vi "StatorResistanceEstimation.vi"(11 "nameplate information":T1) -> (3 "stator resisitance [ohms]":dbl)   [LabVIEW 2017, in "McsaAnalysisFunctions.lvlib"]
doc: "Estimates motor stator resistance based on nameplate information."
uses:
  <vilib>/addons/InsightCM/Utilities/Analysis/MCSA/McsaAnalysisFunctions.lvlib
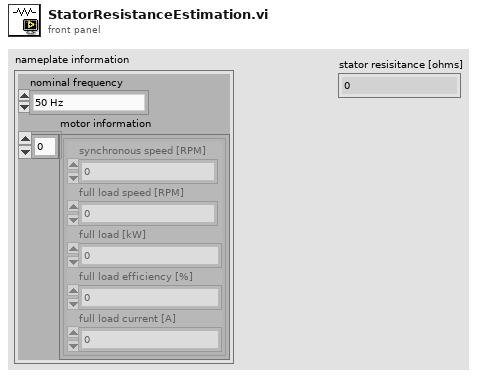
[diagram p1: front panel]
types:
  T1 = cluster{"nominal frequency":enum16{"50 Hz", "60 Hz"}, "motor information":cluster{"synchronous speed [RPM]":dbl, "full load speed [RPM]":dbl, "full load [kW]":dbl, "full load efficiency [%]":dbl, "full load current [A]":dbl}[]}
  T2 = cluster{"synchronous speed [RPM]":dbl, "full load speed [RPM]":dbl, "full load [kW]":dbl, "full load efficiency [%]":dbl, "full load current [A]":dbl}[]
  T3 = cluster{"synchronous speed [RPM]":dbl, "full load speed [RPM]":dbl, "full load [kW]":dbl, "full load efficiency [%]":dbl, "full load current [A]":dbl}
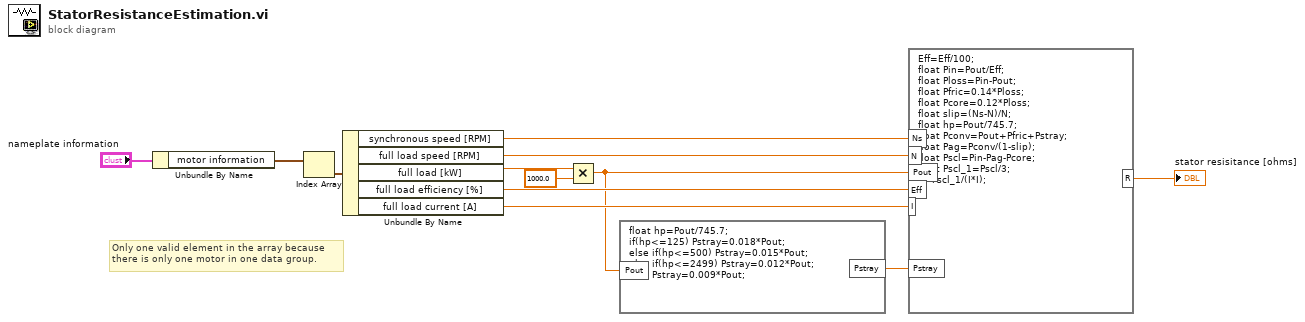
[diagram p0: block diagram]
diagram:
  # "Only one valid element in the array because\nthere is only one motor in one data group."
  n1 = Unbundle By Name("nameplate information") -> ("motor information"=w3:T2)
  n2 = Index Array(array=w3) -> (element=w2:T3)  [unwired: 1 in]
  n3 = Unbundle By Name(w2) -> ("synchronous speed [RPM]"=w10:dbl, "full load speed [RPM]"=w9:dbl, "full load [kW]"=w11:dbl, "full load efficiency [%]"=w6:dbl, "full load current [A]"=w8:dbl)
  n4 = Multiply(x=w11, y=1000.0) -> (x*y=w5:dbl)
  n5 = formula code="float hp=Pout/745.7;\nif(hp<=125) Pstray=0.018*Pout;\nelse if(hp<=500) Pstray=0.015*Pout;\nelse if(hp<=2499) Pstray=0.012*Pout;\nelse Pstray=0.009*Pout;"("Pout"=w5) -> ("Pstray"=w7:dbl)
  n6 = formula code="Eff=Eff/100;\nfloat Pin=Pout/Eff;\nfloat Ploss=Pin-Pout;\nfloat Pfric=0.14*Ploss;\nfloat Pcore=0.12*Ploss;\nfloat slip=(Ns-N)/N;\nfloat hp=Pout/745.7;\nfloat Pconv=Pout+Pfric+Pstray;\nfloat Pag=Pconv/(1-slip);\nfloat Pscl=Pin-Pag-Pcore;\nfloat Pscl_1=Pscl/3;\nR=Pscl_1/(I*I);"("Pout"=w5, "Ns"=w10, "N"=w9, "Eff"=w6, "I"=w8, "Pstray"=w7) -> ("R"=→"stator resisitance [ohms]":dbl)
